vi "mtg demo.vi"() -> ()   [LabVIEW 2025]
uses:
  mtg - action.ctl
panel:
  out "Numeric 10":dbl
  out "Numeric 9":dbl
  out "Numeric 8":dbl
  out "Numeric 7":dbl
  out "Numeric 6":dbl
  out "Numeric 5":dbl
  out "Numeric 4":dbl
  out "Numeric 3":dbl
  out "Numeric 2":dbl
  out "Numeric 1":dbl
  in  "graph selection":T1(ring)
  in  "stop":bool
  out "Chart":dbl[][](graph)
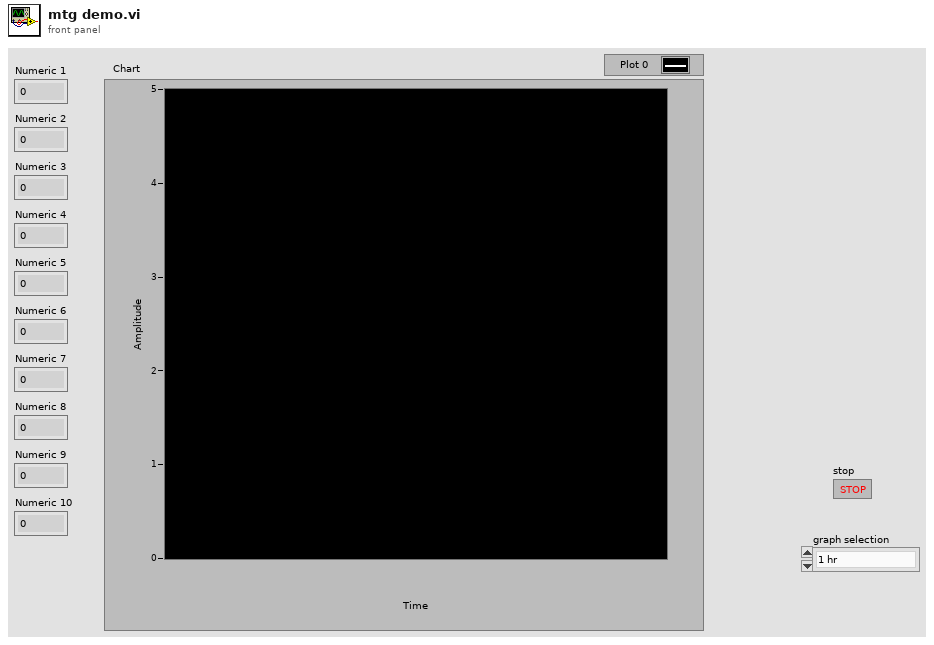
[diagram p1: front panel]
types:
  T1 = enum16{"1 hr", "5 hr", "30 hr", "60 hr", "120 hr", "1 hr (from file)"}
  T2 = typedef "mtg - action.ctl" = enum16{"init", "update data", "change timescale", "get data for file", "get final data for file", "set data from file"}
  T3 = cluster{"session start":path, "seconds in the hour":i32}
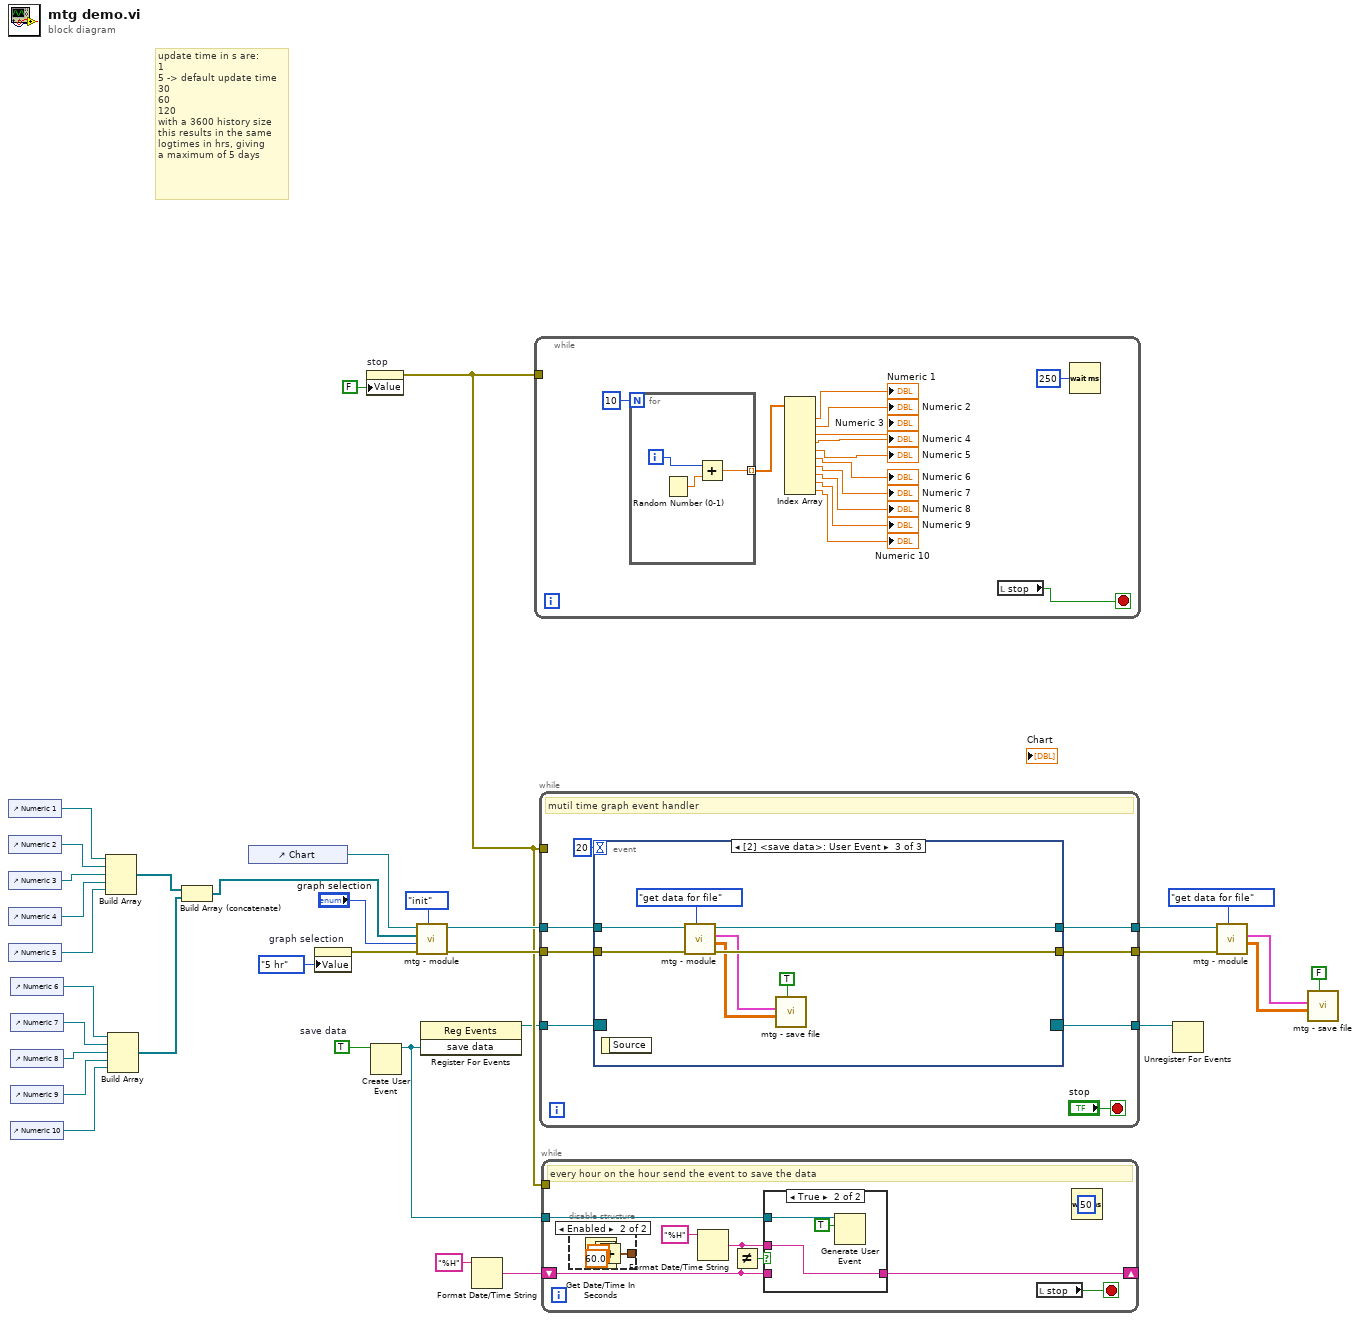
[diagram p0: block diagram]
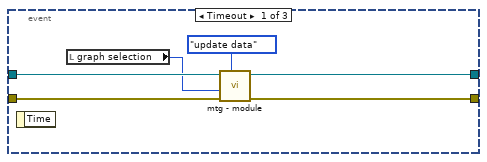
[diagram p4: hidden frame]
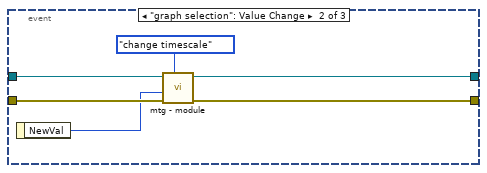
[diagram p5: hidden frame]
diagram:
  w22 = TRUE  # save data
  # "update time in s are:\n1\n5 -> default update time\n30\n60\n120\nwith a 3600 history size\nthis results in the same\nlogtimes in hrs, giving\na maximum of 5 days"
  n1 = control-ref of="Numeric 1"() -> (w34:refnum<vi>)
  n2 = control-ref of="Numeric 2"() -> (w33:refnum<vi>)
  n3 = control-ref of="Numeric 3"() -> (w32:refnum<vi>)
  n4 = control-ref of="Numeric 4"() -> (w31:refnum<vi>)
  n5 = control-ref of="Numeric 5"() -> (w30:refnum<vi>)
  n6 = control-ref of="Numeric 6"() -> (w4:refnum<vi>)
  n7 = control-ref of="Numeric 7"() -> (w5:refnum<vi>)
  n8 = control-ref of="Numeric 8"() -> (w6:refnum<vi>)
  n9 = control-ref of="Numeric 9"() -> (w7:refnum<vi>)
  n10 = control-ref of="Numeric 10"() -> (w8:refnum<vi>)
  n11 = Build Array(w34, w33, w32, w31, w30) -> (w3:refnum<vi>[])
  n12 = Build Array(w4, w5, w6, w7, w8) -> (w2:refnum<vi>[])
  n13 = Build Array (concatenate)(w3, w2) -> (w1:refnum<vi>[])
  n14 = control-ref of="Chart"() -> (w26:refnum<vi>)
  n15 = property on="graph selection" class="Enum (strict)"("Value"=T1."5 hr" ("graph selection")) -> (error out=w23:errorcluster)  [unwired: 2 in, 1 out]
  n16 = property on="stop" class="Bool (strict)"("Value"=FALSE ("stop")) -> (error out=w20:errorcluster)  [unwired: 2 in, 1 out]
  n17 = Create User Event(user event datatype=w22) -> (user event=w16:refnum<user-event>)  [unwired: 1 in, 1 out]
  n18 = call "mtg - module.vi"("action"=mtg_-_action."init", "error in (no error)"=w23, "graph selection"="graph selection", "value references"=w1, "chart in"=w26) -> ("error out"=w27:errorcluster, "chart out"=w28:refnum<vi>)  [unwired: 3 in, 2 out]
  n19 = register-events(w16) -> (reference out=w17:refnum<event-registration>)  [unwired: 2 in, 1 out]
  n20 = Format Date/Time String(time format string (%c)="%H") -> (date/time string=w19:string)  [unwired: 2 in]
  n21 = while {
    tunnel: w20 -> [_]
    stop <- w48 stop-if-true
    n22 = for {
      N: 10 -> [_]
      tunnel: [w49] -> w45 mode=indexing
      i -> [w50]
      n23 = Random Number (0-1)() -> (number: 0 to 1=w51:dbl)
      n24 = Add(x=w50, y=w51) -> (x+y=w49:dbl)
    }
    n25 = Index Array(array=w45) -> (element #1=→"Numeric 1":dbl, element #2=→"Numeric 2":dbl, element #3=→"Numeric 3":dbl, element #4=→"Numeric 4":dbl, element #5=→"Numeric 5":dbl, element #6=→"Numeric 6":dbl, element #7=→"Numeric 7":dbl, element #8=→"Numeric 8":dbl, element #9=→"Numeric 9":dbl, element #10=→"Numeric 10":dbl)  [unwired: 10 in]
    n26 = local read "stop"() -> (w48:bool)
    n27 = Wait (ms)(milliseconds to wait=u32 250) -> ()  [unwired: 1 out]
  }
  n28 = while {
    tunnel: w28 -> [w58]
    tunnel: w27 -> [w57]
    tunnel: [w56] -> w13
    tunnel: [w55] -> w12
    tunnel: w20 -> [_]
    tunnel: w17 -> [w53]
    tunnel: [w52] -> w21
    stop <- "stop" stop-if-true
    # "mutil time graph event handler"
    n29 = event shown="[2] <save data>: User Event" {
      selector: w53 -> [_ _ _]
      dyn-events: [_ _ _] -> w52
      timeout: 20 -> [_ _ _]
      tunnel: w58 -> [w65 w71 w79]
      tunnel: w57 -> [w64 w70 w77]
      tunnel: [w63 w68 w78] -> w56
      tunnel: [w62 w67 w76] -> w55
      event Timeout {
        n30 = event-data() -> ()  [unwired: 1 in, 1 out]
        n31 = local read "graph selection"() -> (w61:T1)
        n32 = call "mtg - module.vi"("action"=mtg_-_action."update data", "error in (no error)"=w64, "graph selection"=w61, "chart in"=w65) -> ("error out"=w62:errorcluster, "chart out"=w63:refnum<vi>)  [unwired: 4 in, 2 out]
      }
      event "graph selection": Value Change {
        n33 = event-data() -> ("NewVal"=w69:T1)  [unwired: 1 in]
        n34 = call "mtg - module.vi"("action"=mtg_-_action."change timescale", "error in (no error)"=w70, "graph selection"=w69, "chart in"=w71) -> ("error out"=w67:errorcluster, "chart out"=w68:refnum<vi>)  [unwired: 4 in, 2 out]
      }
      event User Event {
        n35 = event-data() -> ()  [unwired: 1 in, 1 out]
        n36 = call "mtg - module.vi"("action"=mtg_-_action."get data for file", "error in (no error)"=w77, "chart in"=w79) -> ("error out"=w76:errorcluster, "1 hr History Data"=w73:dbl[][], "date time info"=w74:T3, "chart out"=w78:refnum<vi>)  [unwired: 5 in]
        n37 = call "mtg - save file.vi"("hourly file?"=TRUE, "history data"=w73, "date time info"=w74) -> ()  [unwired: 9 in]
      }
    }
  }
  n38 = while {
    tunnel: w20 -> [_]
    shift-right: [w82] -> _
    shift-left: w19 -> [w81]
    tunnel: w16 -> [w80]
    stop <- w87 stop-if-true
    # "every hour on the hour send the event to save the data"
    n39 = disable-structure shown="Enabled" {
      disable-tunnel: [_ w88] -> _
      frame Disabled {
      }
      frame Enabled {
        n40 = Get Date/Time In Seconds() -> (seconds since 1Jan1904=w91:timestamp)
        n41 = Multiply(x=60.0 ("y"), y=18.0) -> (x*y=w92:dbl)
        n42 = Add(x=w91, y=w92) -> (x+y=w88:timestamp)
      }
    }
    n43 = Format Date/Time String(time format string (%c)="%H") -> (date/time string=w83:string)  [unwired: 2 in]
    n44 = Not Equal?(x=w83, y=w81) -> (x != y?=w84:bool)
    n45 = case shown="True" w84 {
      tunnel: w83 -> [_ w96]
      tunnel: [w93 w96] -> w82
      tunnel: w81 -> [w93 _]
      tunnel: w80 -> [_ w95]
      frame False {
      }
      frame True {
        n46 = Generate User Event(user event=w95, event data cluster=TRUE ("event data")) -> ()  [unwired: 2 in, 2 out]
      }
    }
    n47 = local read "stop"() -> (w87:bool)
    n48 = Wait (ms)(milliseconds to wait=u32 50) -> ()  [unwired: 1 out]
  }
  n49 = Unregister For Events(event registration refnum=w21) -> ()  [unwired: 1 in, 1 out]
  n50 = call "mtg - module.vi"("action"=mtg_-_action."get data for file", "error in (no error)"=w12, "chart in"=w13) -> ("1 hr History Data"=w10:dbl[][], "date time info"=w9:T3)  [unwired: 5 in, 2 out]
  n51 = call "mtg - save file.vi"("hourly file?"=FALSE, "history data"=w10, "date time info"=w9) -> ()  [unwired: 9 in]
